vi "Status.vi"(7 "模式":enum16{"select", "insert", "update", "delete"}(ring), 10 "nameData":cluster{"name":string, "data":string}[](array[cluster])) -> (2 "元素":T1)   [LabVIEW 2013]
uses:
  <vilib>/addons/database/_DB Variant To Data/Database Variant To Data.xnode
panel:
  out "SQL query":string
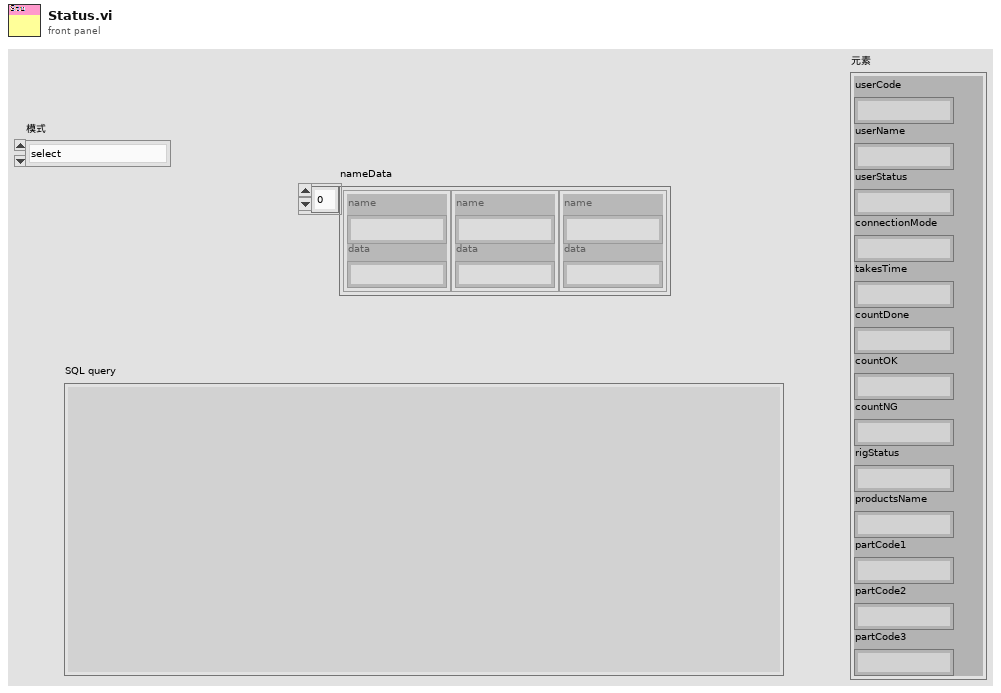
[diagram p1: front panel]
types:
  T1 = cluster{"userCode":string, "userName":string, "userStatus":string, "connectionMode":string, "takesTime":string, "countDone":string, "countOK":string, "countNG":string, "rigStatus":string, "productsName":string, "partCode1":string, "partCode2":string, "partCode3":string}
  T2 = cluster{"userCode":string, "userName":string, "userStatus":string, "connectionMode":string, "takesTime":string, "countDone":string, "countOK":string, "countNG":string, "rigStatus":string, "productsName":string, "partCode1":string, "partCode2":string, "partCode3":string}[]
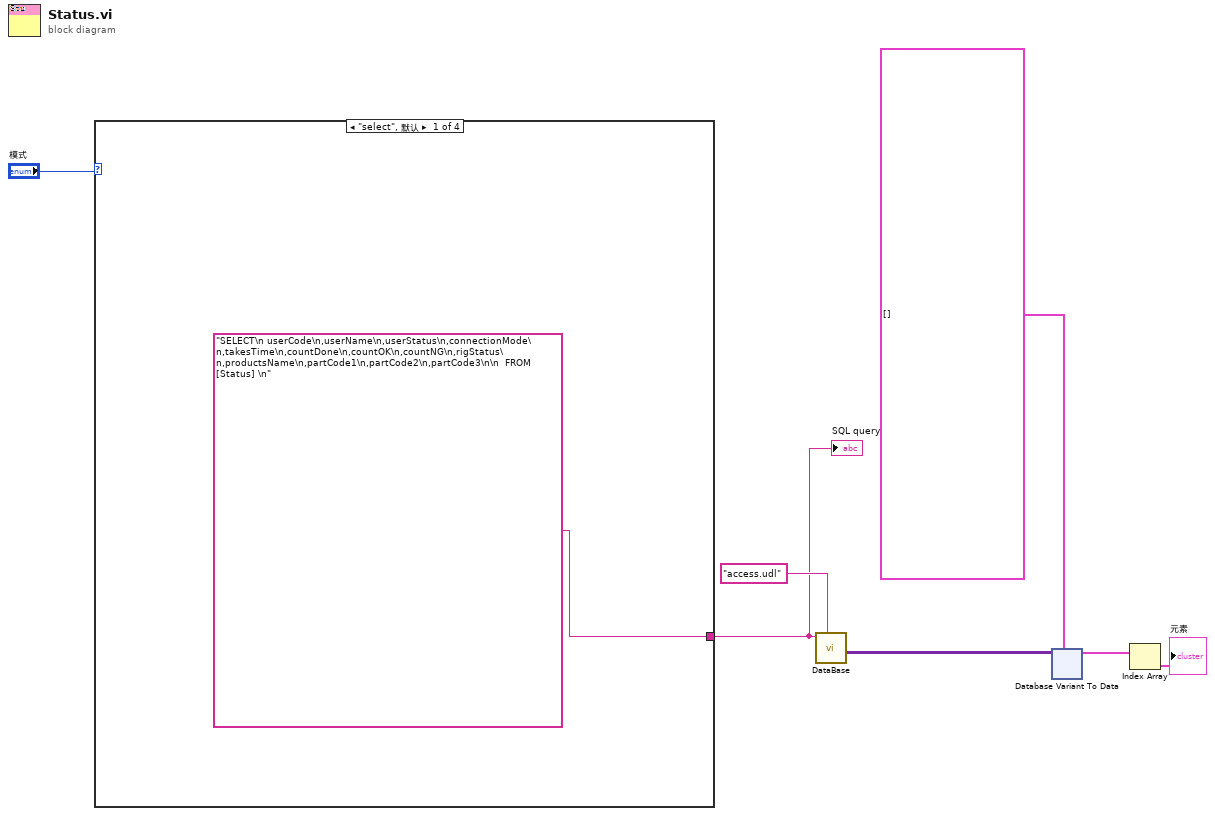
[diagram p0: block diagram]
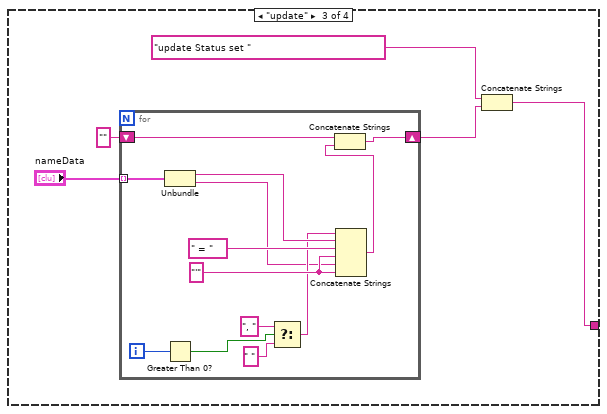
[diagram p3: hidden frame]
diagram:
  n1 = case shown="\"select\", 默认" "模式" {
    tunnel: ["SELECT\n userCode\n,userName\n,userStatus\n,connectionMode\n,takesTime\n,countDone\n,countOK\n,countNG\n,rigStatus\n,productsName\n,partCode1\n,partCode2\n,partCode3\n\n  FROM [Status] \n" ("SQL query") _ w10 _] -> w4
    frame "select", Default {
    }
    frame "insert" {
    }
    frame "update" {
      n2 = for {
        tunnel: "nameData" -> [w26] mode=indexing
        shift-right: [w24] -> w11
        shift-left: "" -> [w25]
        i -> [w23]
        w19 = "'" ("字符串")
        n3 = Unbundle(w26) -> ("name"=w17:string, "data"=w15:string)
        n4 = Greater Than 0?(x=w23) -> (x > 0?=w20:bool)
        n5 = Select(t=", " ("字符串"), s=w20, f=" " ("字符串")) -> (s? t:f=w16:string)
        n6 = Concatenate Strings(w16, w17, " = " ("SQL query"), w19, w15, w19) -> (w14:string)
        n7 = Concatenate Strings(w25, w14) -> (w24:string)
      }
      n8 = Concatenate Strings("update Status set " ("SQL query"), w11) -> (w10:string)
    }
    frame "delete" {
    }
  }
  "SQL query" <- w4
  n9 = call "DataBase.vi"("udl名称"="access.udl", "SQL query"=w4) -> ("recordset data"=w7:variant[][])  [unwired: 9 in]
  n10 = xnode ("Database Variant To Data")("database variant"=w7, "type"=T2 [] ("添加的数组")) -> ("data"=w2:T2)  [unwired: 1 in, 1 out]
  n11 = Index Array(array=w2) -> (element=→"元素":T1)  [unwired: 1 in]
